vi "ServiceChannels.Create.vi"(8 "error in (no error)":errorcluster, 11 "nodeID in":T1 format="%.0x") -> (0 "error out":errorcluster, 3 "nodeID out":u64)   [LabVIEW 2019, in "Diagnostics Addon System Explorer.lvlib"]
uses:
  Diagnostics Addon System Explorer.lvlib
  <vilib>/NI VeriStand/Custom Device API/Custom Device Item Ref.ctl
  <vilib>/NI VeriStand/Custom Device API/Custom Device Channel.ctl
  <vilib>/NI VeriStand/Custom Device API/Custom Device Channel Type.ctl
  Shared/SubVIs/Constants.vi
  <vilib>/NI/NI VeriStand Advanced SysDef API/SysDef API/Advanced System Definition.lvlib
  Shared/Diagnostics Addon Shared.lvlib
  <vilib>/NI VeriStand/Custom Device API/Custom Device API.lvlib
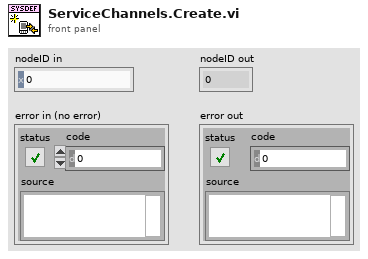
[diagram p1: front panel]
types:
  T1 = typedef "Custom Device API.lvlib/Custom Device Item Ref.ctl" = u64
  T2 = typedef "Custom Device API.lvlib/Custom Device Channel.ctl" = cluster{"Type":T3, "Units":string, "Default Value":dbl, "Faultable":bool, "Scalable":bool}
  T3 = typedef "Custom Device API.lvlib/Custom Device Channel Type.ctl" = enum16{"Input", "Output"}
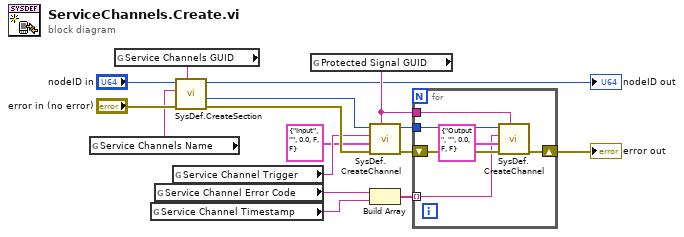
[diagram p0: block diagram]
diagram:
  n1 = global read "Constants.vi" "Service Channels Name"() -> (w1:string)
  n2 = global read "Constants.vi" "Service Channels GUID"() -> (w5:string)
  n3 = global read "Constants.vi" "Service Channel Timestamp"() -> (w7:string)
  n4 = global read "Constants.vi" "Service Channel Error Code"() -> (w6:string)
  n5 = global read "Constants.vi" "Service Channel Trigger"() -> (w10:string)
  n6 = call <vilib>:"SysDef.CreateSection.vi"("GUID"=w5, "error in (no error)"="error in (no error)", "Name"=w1, "nodeID"="nodeID in") -> ("error out"=w14:errorcluster, "New NodeID"=w16:u64, "nodeID out"=→"nodeID out":u64)  [unwired: 4 in, 1 out]
  n7 = global read "Constants.vi" "Protected Signal GUID"() -> (w13:string)
  n8 = call <vilib>:"SysDef.CreateChannel.vi"("GUID"=w13, "error in (no error)"=w14, "Channel"=T2 {"Type"=enum."Input", "Units"="", "Default Value"=0.0, "Faultable"=FALSE, "Scalable"=FALSE}, "Name"=w10, "nodeID"=w16) -> ("error out"=w11:errorcluster, "nodeID out"=w12:u64)  [unwired: 3 in, 2 out]
  n9 = Build Array(w6, w7) -> (w8:string[])
  n10 = for {
    tunnel: w12 -> [w20]
    shift-right: [w19] -> w15
    shift-left: w11 -> [w21]
    tunnel: w8 -> [w18] mode=indexing
    tunnel: w13 -> [w17]
    n11 = call <vilib>:"SysDef.CreateChannel.vi"("GUID"=w17, "error in (no error)"=w21, "Channel"=T2 {"Type"=enum."Output", "Units"="", "Default Value"=0.0, "Faultable"=FALSE, "Scalable"=FALSE}, "Name"=w18, "nodeID"=w20) -> ("error out"=w19:errorcluster)  [unwired: 3 in, 3 out]
  }
  "error out" <- w15
